vi "ChainOfResponsibility1_Main.vi"() -> (0 "error out":errorcluster)   [LabVIEW 2020]
uses:
  SubtractionHandler_class/SubtractionHandler.lvclass
  C:/Projects/DesignPatterns/ChainOfResponsibility1/IHandler_interface/IHandler.lvclass
  C:/Projects/DesignPatterns/ChainOfResponsibility1/BaseHandler_class/BaseHandler.lvclass
  MultiplicationHandler_class/MultiplicationHandler.lvclass
  AdditionHandler_class/AdditionHandler.lvclass
  BaseHandler_class/BaseHandler.lvclass
panel:
  out "Array":dbl[](array[numeric])
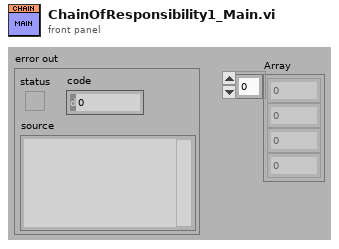
[diagram p1: front panel]
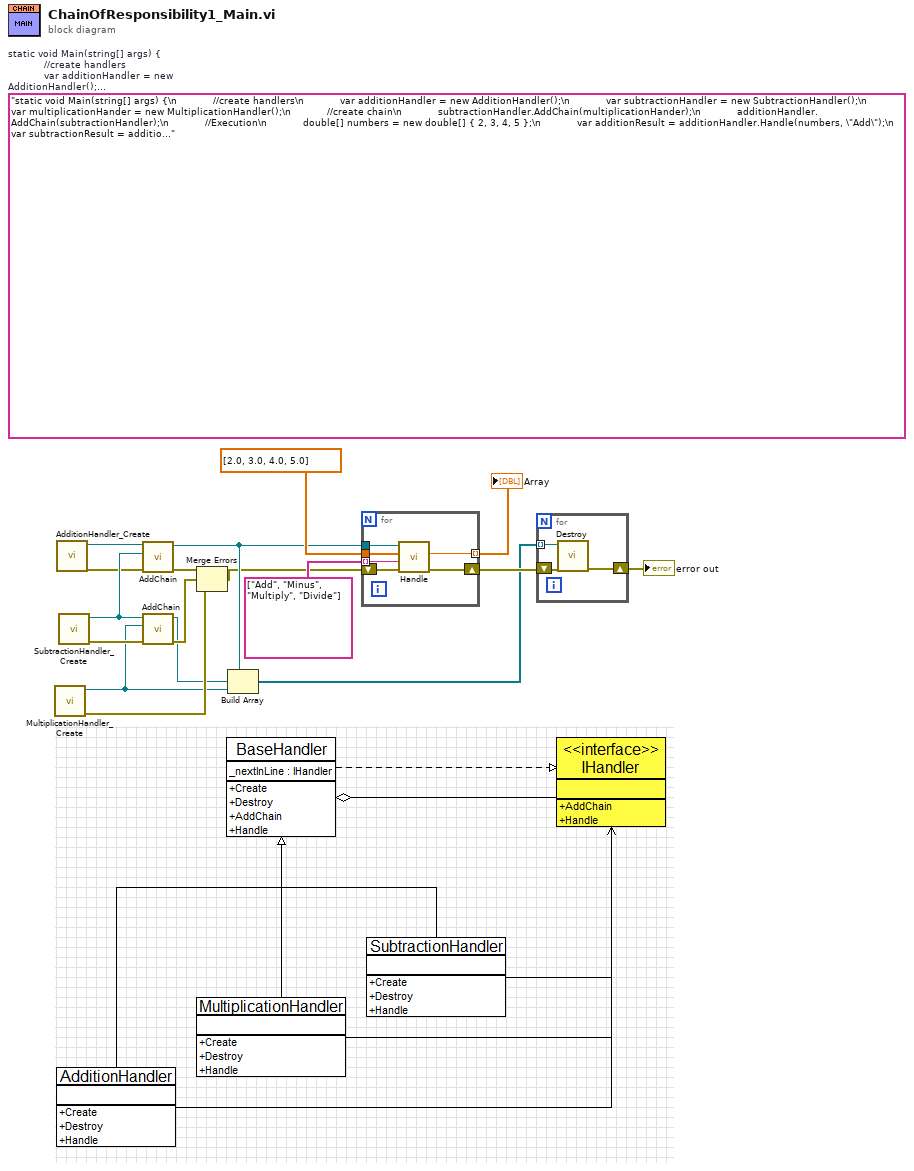
[diagram p0: block diagram]
diagram:
  (unwired) "static void Main(string[] args) {\n            //create handlers\n            var additionHandler = new AdditionHandler();\n            var subtractionHandler = new SubtractionHandler();\n            var multiplicationHander = new MultiplicationHandler();\n            //create chain\n            subtractionHandler.AddChain(multiplicationHander);\n            additionHandler.AddChain(subtractionHandler);\n            //Execution\n            double[] numbers = new double[] { 2, 3, 4, 5 };\n            var additionResult = additionHandler.Handle(numbers, \"Add\");\n            var subtractionResult = additionHandler.Handle(numbers, \"Minus\");\n            var multResult = additionHandler.Handle(numbers, \"Multiply\");\n            var divisionResult = additionHandler.Handle(numbers, \"divide\"); // Divide is not in the chain!!!\n\n            Console.WriteLine(\"Addition = {0}\",additionResult);\n            Console.WriteLine(\"Subtraction = {0}\", subtractionResult);\n            Console.WriteLine(\"Multiplication = {0}\", multResult);\n            Console.WriteLine(\"Division = {0}\", divisionResult);\n        }"  # static void Main(string[] args) {             //create handlers             var additionHandler = new AdditionHandler();             var subtractionHandler = new SubtractionHandler();             var multiplicationHander = new MultiplicationHandler();             //create chain             subtractionHandler.AddChain(multiplicationHander);             additionHandler.AddChain(subtractionHandler);             //Execution             double[] numbers = new double[] { 2, 3, 4, 5 };             var additionResult = additionHandler.Handle(numbers, "Add");             var subtractionResult = additionHandler.Handle(numbers, "Minus");             var multResult = additionHandler.Handle(numbers, "Multiply");             var divisionResult = additionHandler.Handle(numbers, "divide"); // Divide is not in the chain!!!              Console.WriteLine("Addition = {0}",additionResult);             Console.WriteLine("Subtraction = {0}", subtractionResult);             Console.WriteLine("Multiplication = {0}", multResult);             Console.WriteLine("Division = {0}", divisionResult);         }
  n1 = call "MultiplicationHandler_Create.vi"() -> ("Error Out"=w11:errorcluster, "reference out"=w9:refnum<class "MultiplicationHandler.lvclass">)  [unwired: 10 in]
  n2 = call "AdditionHandler_Create.vi"() -> ("Error Out"=w14:errorcluster, "reference out"=w1:refnum<class "AdditionHandler.lvclass">)  [unwired: 10 in]
  n3 = call "SubtractionHandler_Create.vi"() -> ("Error Out"=w12:errorcluster, "reference out"=w17:refnum<class "SubtractionHandler.lvclass">)  [unwired: 10 in]
  n4 = call-dynamic "AddChain.vi"("Error In"=w14, "Handler"=w17, "reference in"=w1) -> ("Error Out"=w4:errorcluster, "reference out"=w7:refnum<class "AdditionHandler.lvclass">)  [unwired: 7 in]
  n5 = call-dynamic "AddChain.vi"("Error In"=w12, "Handler"=w9, "reference in"=w17) -> ("Error Out"=w13:errorcluster, "reference out"=w8:refnum<class "SubtractionHandler.lvclass">)  [unwired: 7 in]
  n6 = Merge Errors(w4, w13, w11) -> (w3:errorcluster)
  n7 = Build Array(w7, w8, w9) -> (w6:refnum<class "BaseHandler.lvclass">[])
  n8 = for {
    tunnel: w7 -> [w23]
    tunnel: dbl[] [2.0, 3.0, 4.0, 5.0] -> [w22]
    tunnel: string[] ["Add", "Minus", "Multiply", "Divide"] -> [w21] mode=indexing
    shift-right: [w19] -> w10
    shift-left: w3 -> [w20]
    tunnel: [w18] -> w2 mode=indexing
    n9 = call-dynamic "Handle.vi"("Error In"=w20, "Action"=w21, "Values"=w22, "reference in"=w23) -> ("Error Out"=w19:errorcluster, "Return(DBL)"=w18:dbl)  [unwired: 5 in, 1 out]
  }
  "Array" <- w2
  n10 = for {
    tunnel: w6 -> [w25] mode=indexing
    shift-right: [w24] -> w5
    shift-left: w10 -> [w26]
    n11 = call-dynamic "Destroy.vi"("Error In"=w26, "reference in"=w25) -> ("Error Out"=w24:errorcluster)  [unwired: 8 in, 1 out]
  }
  "error out" <- w5
